vi "Configure Datafinder for Spartan.vi"(8 "error in (no error)":errorcluster, 11 "Data Path":path) -> (0 "error out":errorcluster)   [LabVIEW 2011]
uses:
  <vilib>/Utility/sysdir.llb/System Directory Type.ctl
panel:
  out "PROBE:  New Config":string
  out "PROBE:  Original Config":string
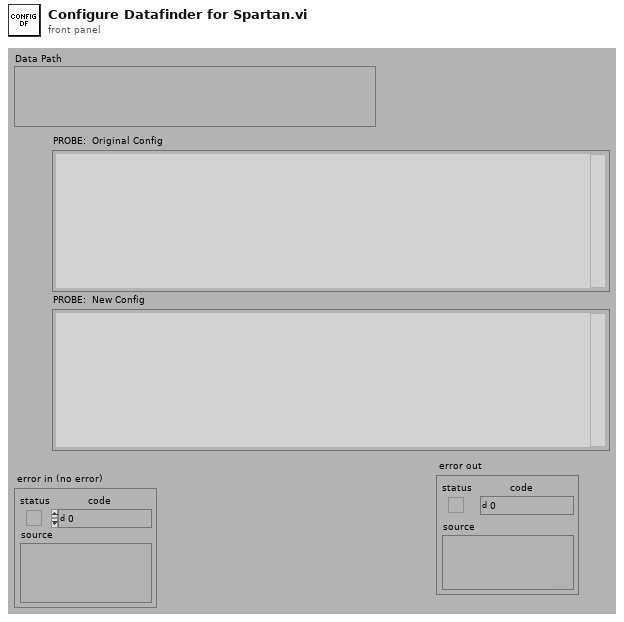
[diagram p1: front panel]
types:
  T1 = typedef "System Directory Type.ctl" = i32
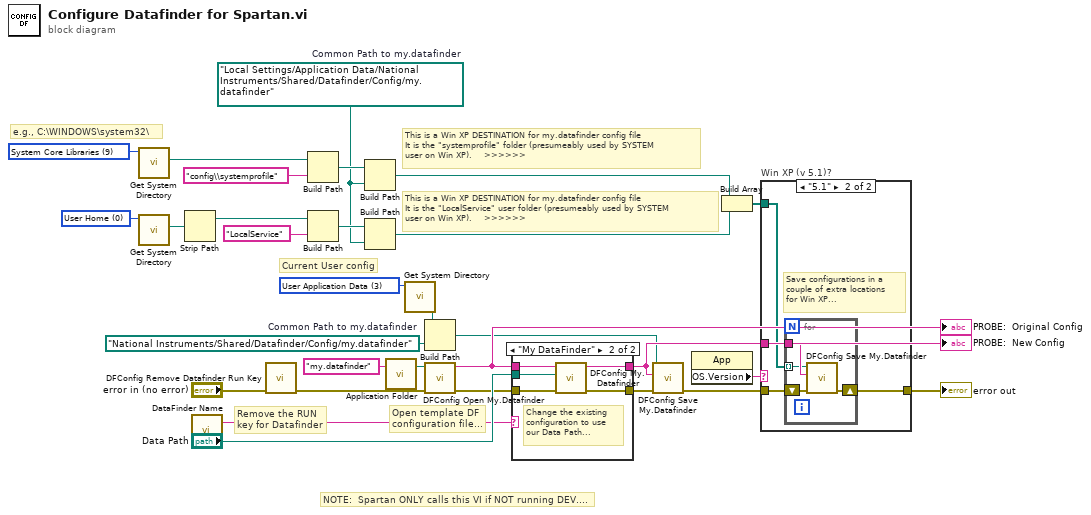
[diagram p0: block diagram]
diagram:
  w5 = path "National Instruments/Shared/Datafinder/Config/my.datafinder"  # Common Path to my.datafinder
  w7 = T1 3 items=["User Home", "User Desktop", "User Documents", "User Application Data", "User Preferences", "User Temporary", "Public Documents", "Public Application Data", "Public Preferences", "System Core Libraries", "System Installed Libraries", "Application Files", "Boot Volume Root"] ("system directory type")
  w18 = T1 0 items=["User Home", "User Desktop", "User Documents", "User Application Data", "User Preferences", "User Temporary", "Public Documents", "Public Application Data", "Public Preferences", "System Core Libraries", "System Installed Libraries", "Application Files", "Boot Volume Root"] ("system directory type")
  w22 = T1 9 items=["User Home", "User Desktop", "User Documents", "User Application Data", "User Preferences", "User Temporary", "Public Documents", "Public Application Data", "Public Preferences", "System Core Libraries", "System Installed Libraries", "Application Files", "Boot Volume Root"] ("system directory type")
  w14 = path "Local Settings/Application Data/National Instruments/Shared/Datafinder/Config/my.datafinder"  # Common Path to my.datafinder
  # "Open template DF\nconfiguration file..."
  # "This is a Win XP DESTINATION for my.datafinder config file\nIt is the \"LocalService\" user folder (presumeably used by SYSTEM\nuser on Win XP).    >>>>>>"
  # "e.g., C:\\WINDOWS\\system32\\"
  # "This is a Win XP DESTINATION for my.datafinder config file\nIt is the \"systemprofile\" folder (presumeably used by SYSTEM\nuser on Win XP).    >>>>>>"
  # "Current User config"
  # "Remove the RUN\nkey for Datafinder"
  # "NOTE:  Spartan ONLY calls this VI if NOT running DEV...."
  n1 = call <vilib>:"Get System Directory.vi"("system directory type"=w22) -> ("system directory"=w21:path)  [unwired: 10 in]
  n2 = call <vilib>:"Get System Directory.vi"("system directory type"=w18) -> ("system directory"=w17:path)  [unwired: 10 in]
  n3 = Strip Path(path=w17) -> (stripped path=w4:path)  [unwired: 1 out]
  n4 = call "DataFinder Name.vi"() -> ("DataFinder Name"=w25:string)  [unwired: 3 in]
  n5 = call "DFConfig Remove Datafinder Run Key.vi"("error in (no error)"="error in (no error)") -> ("error out"=w24:errorcluster)  [unwired: 10 out]
  n6 = Build Path(base path=w21, name or relative path="config\\systemprofile" ("Path")) -> (appended path=w19:path)
  n7 = Build Path(base path=w4, name or relative path="LocalService" ("Path")) -> (appended path=w15:path)
  n8 = Build Path(base path=w19, name or relative path=w14) -> (appended path=w13:path)
  n9 = Build Path(base path=w15, name or relative path=w14) -> (appended path=w12:path)
  n10 = call "Application Folder.vi"("Relative Path (\"\" - Folder)"="my.datafinder") -> ("Application Folder"=w3:path)  [unwired: 2 in]
  n11 = call <vilib>:"Get System Directory.vi"("system directory type"=w7) -> ("system directory"=w6:path)  [unwired: 10 in]
  n12 = Build Path(base path=w6, name or relative path=w5) -> (appended path=w1:path)
  n13 = call "DFConfig Open My.Datafinder.vi"("error in (no error)"=w24, "my.datafinder Path (empty)"=w3) -> ("error out"=w23:errorcluster, "my.datafinder"=w27:string)  [unwired: 8 out]
  "PROBE:  Original Config" <- w27
  n14 = case shown="\"My DataFinder\"" w25 {
    tunnel: "Data Path" -> [_ w37]
    tunnel: w23 -> [w32 w36]
    tunnel: w27 -> [w31 w35]
    tunnel: [w31 w34] -> w26
    tunnel: [w32 w33] -> w8
    frame Default {
    }
    frame "My DataFinder" {
      # "Change the existing\nconfiguration to use\nour Data Path..."
      n15 = call "DFConfig My.Datafinder.vi"("error in (no error)"=w36, "Spartan Data Path (\"\")"=w37, "My.DataFinder In"=w35) -> ("error out"=w33:errorcluster, "My.DataFinder Out"=w34:string)  [unwired: 2 in, 5 out]
    }
  }
  "PROBE:  New Config" <- w26
  n16 = call "DFConfig Save My.Datafinder.vi"("error in (no error)"=w8, "my.datafinder (\"\")"=w26, "my.datafinder Path (empty)"=w1) -> ("error out"=w9:errorcluster)  [unwired: 8 out]
  n17 = property class="App"() -> ("OS.Version"=w10:string)  [unwired: 2 in, 2 out]
  n18 = Build Array(w13, w12) -> (w11:path[])
  n19 = case "Win XP (v 5.1)?" shown="\"5.1\"" w10 {
    tunnel: w9 -> [w38 w41]
    tunnel: [w38 w40] -> w29
    tunnel: w26 -> [_ w42]
    tunnel: w11 -> [_ w39]
    frame Default {
    }
    frame "5.1" {
      # "Save configurations in a\ncouple of extra locations\nfor Win XP..."
      n20 = for {
        tunnel: w42 -> [w46]
        tunnel: w39 -> [w45] mode=indexing
        shift-right: [w43] -> w40
        shift-left: w41 -> [w44]
        n21 = call "DFConfig Save My.Datafinder.vi"("error in (no error)"=w44, "my.datafinder (\"\")"=w46, "my.datafinder Path (empty)"=w45) -> ("error out"=w43:errorcluster)  [unwired: 8 out]
      }
    }
  }
  "error out" <- w29
